vi "NIMS_NS_iir_notch.vi"(5 "Function name":string, 6 "Line number":i32, 7 "Number of outputs requested":i32, 8 "error in (no error)":errorcluster, 11 "[A]":variant[](array[variant])) -> (0 "error out":errorcluster, 3 "[funct(A)]":variant[](array[variant]))   [LabVIEW 2017]
uses:
  <vilib>/imath/engines/lvmath/Functions/Error Handling/error.ctl
  <instcachedir>/0/NIMS_RunTimeType_From StrictType (excl LVString)_1019F277F0A747EDBCA0F6C52CA54500.lvgen/NIMS_RunTimeType_From StrictType (excl LVString)_1019F277F0A747EDBCA0F6C52CA54500_000.vi
  <instcachedir>/0/NIMS_Get Scalar_w Error_1987D997E87247DDAC16EA23A5E9E4FC.lvgen/NIMS_Get Scalar_w Error_1987D997E87247DDAC16EA23A5E9E4FC_003.vi
  <instcachedir>/0/NIMS_Complex To Real_BE01396FDE034E8E94CEBBA1E368668D.lvgen/NIMS_Complex To Real_BE01396FDE034E8E94CEBBA1E368668D_000.vi
  <instcachedir>/0/NIMS_RunTimeType_To Numeric_1CBDAFC4EFAD4045A1DE52278D16738D.lvgen/NIMS_RunTimeType_To Numeric_1CBDAFC4EFAD4045A1DE52278D16738D_000.vi
  <vilib>/addons/Digital Filter Design/NI_DigFilter_MathScript.lvlib
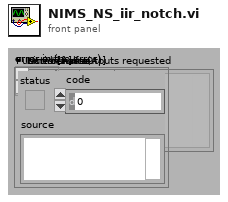
[diagram p1: front panel]
types:
  T1 = typedef "error.ctl" = enum16{"No Error", "Problem", "Input type must not be void", "Incorrect number of parameters", "Function not defined for non-numeric types", "An output variable of the user-defined function is undefined", "Function only defined for character arrays", "Function not defined for boolean, character, or single precision", "Function not defined for complex types", "Not a valid operation", "Inputs must be scalar", "Input matrices are not the same size", "Function only available on RT", "Input matrices must be nonnegative integers of the same type", "Arguments must be non-negative integers less than bitmax", "Number to complement must be less than 2^N", "Bit to get is outside range", "Bit to set is outside range", "Input must be real type ", "At least one parameter must be scalar", "Unable to display plug-in data on RT", "Function not defined for higher dimensional matrices", "Invalid attributes", "Wrong Type of Input Arguments", "Wrong Argument Option", "Invalid file identifier", "Indices must be real positive integers", "The variable is not a matrix data type.", "Number of elements must be the same for indices and values", "You cannot replace elements of a matrix with non-matrix data types.", "Cannot resize a 2D matrix with a linear index", "Unknown variable or symbol", "Indices out of range", "Empty matrix deletion can not be used with two indices", "Number of rows and columns must be the same for indices and values.", "Complex cannot be converted to Boolean", "Char cannot be converted to Boolean", "int64 cannot be converted to Boolean", "uint64 cannot be converted to Boolean", "You cannot convert a Boolean to a character.", "Incompatible input size in 3D surface function", "All rows must have the same number of columns", "Incompatible types", "Invalid matrix dimensions", "Dimension must be 1 or 2", "Base must be an integer between 2 and 36", "Invalid input", "Square matrix required", "Function 'timerstart' must be called before 'timerstop'", "Arguments must be positive real", "Step must not be zero", "Wrong number of input arguments", "Wrong number of output arguments", "Too many index arguments", "Input scalar must be >= 0", "Input scalar must be positive", "Input scalar must not be 0", "Input scalar must be in range [0,1]", "Can't use conditionally defined variable that's undefined", "Input must be a vector", "RT Exec Trace Toolkit not licensed", "Empty vector error", "All elements must be in domain [-1,1]", "All real elements of input vector must be >= 0", "All elements of input vector must be positive", "Values of input vectors are not compatible", "DAQmx not installed", "Input vector must be an increasing vector", "Dereferenced field does not exist within the struct", "A vector or matrix of structures must be indexed before it can be dereferenced", "Lenths of two input vectors are not compatible", "Invalid fieldname", "Empty matrix error", "Cannot use '.' on a type other than Struct", "Unused074", "Data type of the struct's field name is invalid", "Using . to dereference data that is not a struct", "Input struct contains invalid type ", "Size of input matrix is incompatible with input size", "Invalid format specifier", "Could not find field within struct", "Bad permutation array", "Mismatched fieldnames", "ode: User Function could not be opened", "ode: User Function signature does not meet ode requirements", "Unused085", "RunTime: MathScript could not be compiled", "Unknown function", "Only scalars and strings supported", "ode: User Function signature has incorrect number of inputs", "ode:User Function signature has incorrect number of outputs", "Range is too large", "End used without variable", "Function not available (RTE)", "Custom user error", "Arguments must be integers less than bitmax", "Shared library not found", "Header file not found", "Shared library already loaded", "Shared library not loaded", "Shared library function not found", "Shared library string return problem", "Problem calling shared library function", "Problem loading shared library from OS", "Problem parsing shared library header file", "Shared library incompatible types", "Shared library unsupported return type", "Shared library function not exported", "Shared library unsupported input type", "Problem unloading shared library from OS", "Function only available from UI", "Function specified in argument is missing", "An internal error has occurred", "Invalid object", "Invalid property", "Read-only property", "A break command has occurred", "A continue command has occurred", "A return command has occurred", "ode: times parameter invalid", "Function specified in argument has incorrect signature", "Function not found in file", "Reserved keyword cannot be defined as variable", "Reserved keyword cannot be defined as a function or script", "Arguments must be string literals", "Function not supported on this platform", "All columns must have the same number of rows", "Function ignored in RTE warning", "Cannot use : as a parameter that is not a variable", "Output can't be coerced to requested type", "Function not supported on current target", "Variable dependent on an unwired function input", "Unused132", "Unused133", "Unused134", "Unused135", "Unused136", "Unused137", "Unused138", "Unused139", "Global/Persistent must only take constants as arguments.", "Varargin must be last input in the function definition.", "Varargout must be last output in the function definition.", "Invalid output type. Cannot output a cell array of any type other than string.", "Invalid output type. Type is a dynamic struct.", "Invalid output type. Type is a struct that has a field whose type is not known until run-time", "Invalid output type. Type is a struct that has a field which is a plot object.", "MathScript parser DLL missing", "MathScript requires LabVIEW Full", "MathScript license is invalid or missing", "Varargout not supported except in assignments."}
  T2 = typedef "NIMS_CH_character datatype.ctl" = cluster{"Numeric":u8}
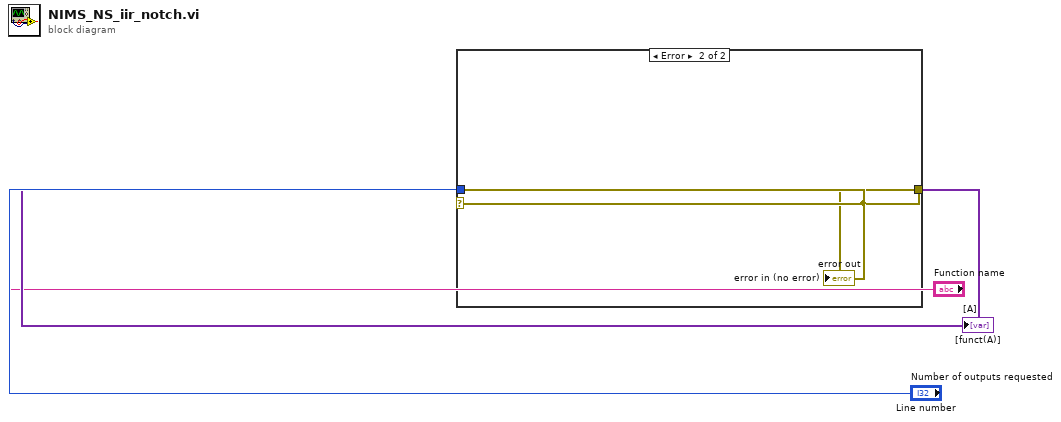
[diagram p0: block diagram]
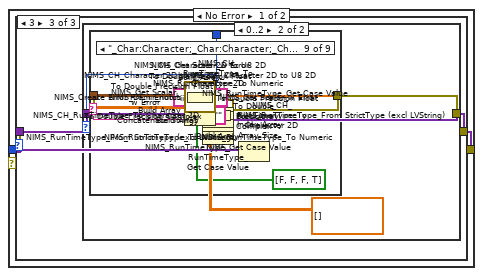
[diagram p2: hidden frame]
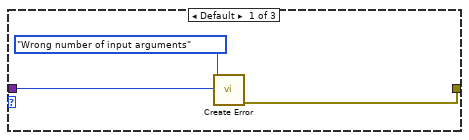
[diagram p3: hidden frame]
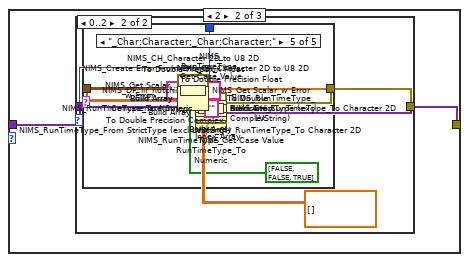
[diagram p4: hidden frame]
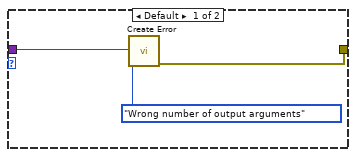
[diagram p5: hidden frame]
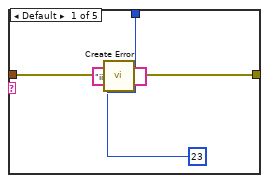
[diagram p6: hidden frame]
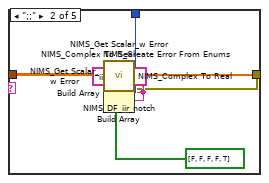
[diagram p7: hidden frame]
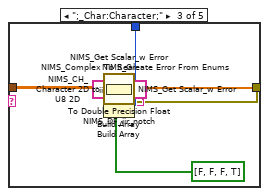
[diagram p8: hidden frame]
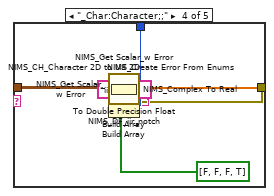
[diagram p9: hidden frame]
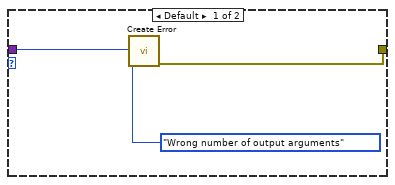
[diagram p10: hidden frame]
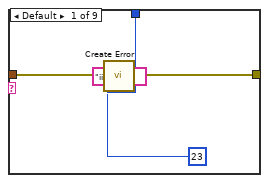
[diagram p11: hidden frame]
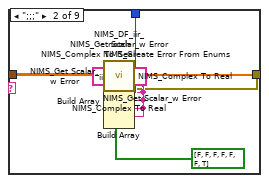
[diagram p12: hidden frame]
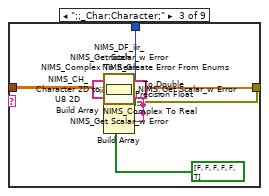
[diagram p13: hidden frame]
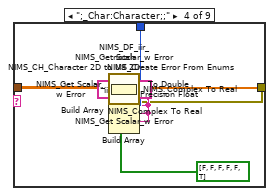
[diagram p14: hidden frame]
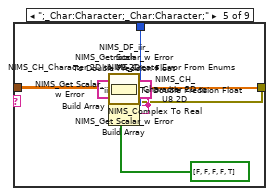
[diagram p15: hidden frame]
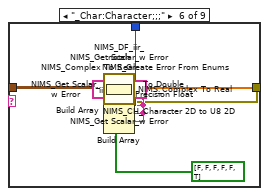
[diagram p16: hidden frame]
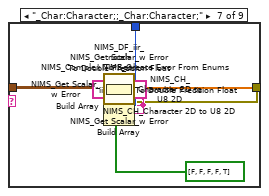
[diagram p17: hidden frame]
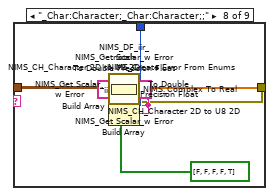
[diagram p18: hidden frame]
diagram:
  n1 = case shown="Error" "error in (no error)" {
    selector: "error in (no error)" -> [_ w404]
    tunnel: [w15 _] -> w4
    tunnel: [w14 w404] -> w3
    tunnel: "error in (no error)" -> [w13 _]
    tunnel: "Number of outputs requested" -> [w12 _]
    tunnel: "[A]" -> [w11 _]
    tunnel: "Function name" -> [w10 _]
    tunnel: "Line number" -> [w9 _]
    frame No Error {
      n2 = Array Size(array=w11) -> (size(s)=w8:i32)
      n3 = case shown="3" w8 {
        tunnel: [_ w27 w154] -> w15
        tunnel: w10 -> [w19 w24 w151]
        tunnel: w9 -> [w20 w25 w152]
        tunnel: w13 -> [w17 w23 w150]
        tunnel: [w16 w22 w149] -> w14
        tunnel: w12 -> [_ w21 w148]
        tunnel: w11 -> [_ w26 w153]
        frame Default {
          n4 = call <vilib>:"Create Error.vi"("Function name"=w19, "error in (no error)"=w17, "Error Enum"=error."Wrong number of input arguments", "Line number"=w20) -> ("error out"=w16:errorcluster)  [unwired: 6 in, 1 out]
        }
        frame 2 {
          n5 = case shown="0..2" w21 {
            tunnel: [_ w33] -> w27
            tunnel: w24 -> [w31 _]
            tunnel: w25 -> [w32 w57]
            tunnel: w23 -> [w29 w55]
            tunnel: [w28 w44] -> w22
            tunnel: w26 -> [_ w58]
            frame Default {
              n6 = call <vilib>:"Create Error.vi"("Function name"=w31, "error in (no error)"=w29, "Error Enum"=error."Wrong number of output arguments", "Line number"=w32) -> ("error out"=w28:errorcluster)  [unwired: 6 in, 1 out]
            }
            frame 0..2 {
              n7 = Index Array(array=w58) -> (element #1=w54:variant, element #2=w49:variant)  [unwired: 2 in]
              n8 = call <vilib>:"NIMS_RunTimeType_Get Case Value.vi"("Data In"=w49) -> ("Case Value"=w45:string)  [unwired: 9 in, 1 out]
              n9 = call <vilib>:"NIMS_CH_RunTimeType_To Character 2D.vi"("Variant"=w49) -> ("data"=w46:T2[][])  [unwired: 1 in]
              n10 = call-generic <vilib>:"NIMS_RunTimeType_To Numeric.vi"("DataType"=cdb[][] [], "Variant"=w49) -> ("data"=w47:cdb[][])  [unwired: 1 in]
              n11 = call <vilib>:"NIMS_RunTimeType_Get Case Value.vi"("Data In"=w54) -> ("Case Value"=w50:string)  [unwired: 9 in, 1 out]
              n12 = call <vilib>:"NIMS_CH_RunTimeType_To Character 2D.vi"("Variant"=w54) -> ("data"=w51:T2[][])  [unwired: 1 in]
              n13 = call-generic <vilib>:"NIMS_RunTimeType_To Numeric.vi"("DataType"=cdb[][] [], "Variant"=w54) -> ("data"=w52:cdb[][])  [unwired: 1 in]
              n14 = Concatenate Strings(w50, w45) -> (w56:string)
              n15 = case shown="\"_Char:Character;_Char:Character;\"" w56 {
                tunnel: w55 -> [w60 w70 w91 w112 w133]
                tunnel: [_ w65 w86 w107 w128] -> w43
                tunnel: [_ w64 w85 w106 w127] -> w39
                tunnel: [w59 w66 w87 w108 w129] -> w44
                tunnel: w52 -> [_ w83 w104 _ _]
                tunnel: w51 -> [_ _ _ w125 w146]
                tunnel: w47 -> [_ w80 _ w121 _]
                tunnel: w46 -> [_ _ w101 _ w142]
                tunnel: w57 -> [w63 w73 w94 w115 w136]
                frame Default {
                  n16 = call <vilib>:"Create Error.vi"("Function name"="iir_notch", "error in (no error)"=w60, "Error Enum"=23, "Line number"=w63) -> ("error out"=w59:errorcluster)  [unwired: 6 in, 1 out]
                }
                frame ";;" {
                  w68 = "iir_notch"
                  n17 = call-generic <vilib>:"NIMS_Complex To Real.vi"("A"=w80) -> ("Error Enum"=w76:T1, "Real(A)"=w79:dbl[][])  [unwired: 8 in, 1 out]
                  n18 = call-generic <vilib>:"NIMS_Get Scalar_w Error.vi"("A"=w79) -> ("Error Enum"=w75:T1, "Scalar"=w81:dbl)  [unwired: 8 in, 1 out]
                  n19 = call-generic <vilib>:"NIMS_Complex To Real.vi"("A"=w83) -> ("Error Enum"=w78:T1, "Real(A)"=w82:dbl[][])  [unwired: 8 in, 1 out]
                  n20 = call-generic <vilib>:"NIMS_Get Scalar_w Error.vi"("A"=w82) -> ("Error Enum"=w77:T1, "Scalar"=w84:dbl)  [unwired: 8 in, 1 out]
                  n21 = call <vilib>:"NIMS_DF_iir_notch.vi"("bw"=w81, "w"=w84) -> ("error"=w74:i32, "a"=w64:dbl[], "b"=w65:dbl[])  [unwired: 7 in]
                  n22 = Build Array(w68, w68, w68, w68, "iir_notch") -> (w71:string[])
                  n23 = Build Array(w78, w77, w76, w75, w74) -> (w72:i32[])
                  n24 = call <vilib>:"NIMS_Create Error From Enums.vi"("Error Code"=bool[] [FALSE, FALSE, FALSE, FALSE, TRUE], "error in (no error)"=w70, "Line no"=w73, "Error Enums"=w72, "Function names"=w71) -> ("error out"=w66:errorcluster)  [unwired: 6 in]
                }
                frame ";_Char:Character;" {
                  w89 = "iir_notch"
                  n25 = call <vilib>:"NIMS_CH_Character 2D to U8 2D.vi"("Character 2D array"=w101) -> ("U8 2D array"=w100:u8[][])  [unwired: 10 in]
                  n26 = To Double Precision Float(number=w100) -> (double precision float=w99:dbl[][])
                  n27 = call-generic <vilib>:"NIMS_Get Scalar_w Error.vi"("A"=w99) -> ("Error Enum"=w96:T1, "Scalar"=w102:dbl)  [unwired: 8 in, 1 out]
                  n28 = call-generic <vilib>:"NIMS_Complex To Real.vi"("A"=w104) -> ("Error Enum"=w98:T1, "Real(A)"=w103:dbl[][])  [unwired: 8 in, 1 out]
                  n29 = call-generic <vilib>:"NIMS_Get Scalar_w Error.vi"("A"=w103) -> ("Error Enum"=w97:T1, "Scalar"=w105:dbl)  [unwired: 8 in, 1 out]
                  n30 = call <vilib>:"NIMS_DF_iir_notch.vi"("bw"=w102, "w"=w105) -> ("error"=w95:i32, "a"=w85:dbl[], "b"=w86:dbl[])  [unwired: 7 in]
                  n31 = Build Array(w89, w89, w89, "iir_notch") -> (w92:string[])
                  n32 = Build Array(w98, w97, w96, w95) -> (w93:i32[])
                  n33 = call <vilib>:"NIMS_Create Error From Enums.vi"("Error Code"=bool[] [FALSE, FALSE, FALSE, TRUE], "error in (no error)"=w91, "Line no"=w94, "Error Enums"=w93, "Function names"=w92) -> ("error out"=w87:errorcluster)  [unwired: 6 in]
                }
                frame "_Char:Character;;" {
                  w110 = "iir_notch"
                  n34 = call-generic <vilib>:"NIMS_Complex To Real.vi"("A"=w121) -> ("Error Enum"=w118:T1, "Real(A)"=w120:dbl[][])  [unwired: 8 in, 1 out]
                  n35 = call-generic <vilib>:"NIMS_Get Scalar_w Error.vi"("A"=w120) -> ("Error Enum"=w117:T1, "Scalar"=w122:dbl)  [unwired: 8 in, 1 out]
                  n36 = call <vilib>:"NIMS_CH_Character 2D to U8 2D.vi"("Character 2D array"=w125) -> ("U8 2D array"=w124:u8[][])  [unwired: 10 in]
                  n37 = To Double Precision Float(number=w124) -> (double precision float=w123:dbl[][])
                  n38 = call-generic <vilib>:"NIMS_Get Scalar_w Error.vi"("A"=w123) -> ("Error Enum"=w119:T1, "Scalar"=w126:dbl)  [unwired: 8 in, 1 out]
                  n39 = call <vilib>:"NIMS_DF_iir_notch.vi"("bw"=w122, "w"=w126) -> ("error"=w116:i32, "a"=w106:dbl[], "b"=w107:dbl[])  [unwired: 7 in]
                  n40 = Build Array(w110, w110, w110, "iir_notch") -> (w113:string[])
                  n41 = Build Array(w119, w118, w117, w116) -> (w114:i32[])
                  n42 = call <vilib>:"NIMS_Create Error From Enums.vi"("Error Code"=bool[] [FALSE, FALSE, FALSE, TRUE], "error in (no error)"=w112, "Line no"=w115, "Error Enums"=w114, "Function names"=w113) -> ("error out"=w108:errorcluster)  [unwired: 6 in]
                }
                frame "_Char:Character;_Char:Character;" {
                  w131 = "iir_notch"
                  n43 = call <vilib>:"NIMS_CH_Character 2D to U8 2D.vi"("Character 2D array"=w142) -> ("U8 2D array"=w141:u8[][])  [unwired: 10 in]
                  n44 = To Double Precision Float(number=w141) -> (double precision float=w140:dbl[][])
                  n45 = call-generic <vilib>:"NIMS_Get Scalar_w Error.vi"("A"=w140) -> ("Error Enum"=w138:T1, "Scalar"=w143:dbl)  [unwired: 8 in, 1 out]
                  n46 = call <vilib>:"NIMS_CH_Character 2D to U8 2D.vi"("Character 2D array"=w146) -> ("U8 2D array"=w145:u8[][])  [unwired: 10 in]
                  n47 = To Double Precision Float(number=w145) -> (double precision float=w144:dbl[][])
                  n48 = call-generic <vilib>:"NIMS_Get Scalar_w Error.vi"("A"=w144) -> ("Error Enum"=w139:T1, "Scalar"=w147:dbl)  [unwired: 8 in, 1 out]
                  n49 = call <vilib>:"NIMS_DF_iir_notch.vi"("bw"=w143, "w"=w147) -> ("error"=w137:i32, "a"=w127:dbl[], "b"=w128:dbl[])  [unwired: 7 in]
                  n50 = Build Array(w131, w131, "iir_notch") -> (w134:string[])
                  n51 = Build Array(w139, w138, w137) -> (w135:i32[])
                  n52 = call <vilib>:"NIMS_Create Error From Enums.vi"("Error Code"=bool[] [FALSE, FALSE, TRUE], "error in (no error)"=w133, "Line no"=w136, "Error Enums"=w135, "Function names"=w134) -> ("error out"=w129:errorcluster)  [unwired: 6 in]
                }
              }
              n53 = Build Array(w39) -> (w38:dbl[][])
              n54 = To Double Precision Complex(1:w38) -> (0:w37:cdb[][])
              n55 = call-generic <vilib>:"NIMS_RunTimeType_From StrictType (excl LVString).vi"("Plug-In Name"="", "Data In"=w37) -> ("Data Out"=w34:variant)  [unwired: 2 in]
              n56 = Build Array(w43) -> (w42:dbl[][])
              n57 = To Double Precision Complex(1:w42) -> (0:w41:cdb[][])
              n58 = call-generic <vilib>:"NIMS_RunTimeType_From StrictType (excl LVString).vi"("Plug-In Name"="", "Data In"=w41) -> ("Data Out"=w35:variant)  [unwired: 2 in]
              n59 = Build Array(w35, w34) -> (w33:variant[])
            }
          }
        }
        frame 3 {
          n60 = case shown="0..2" w148 {
            tunnel: [_ w160] -> w154
            tunnel: w151 -> [w158 _]
            tunnel: w152 -> [w159 w189]
            tunnel: w150 -> [w156 w187]
            tunnel: [w155 w171] -> w149
            tunnel: w153 -> [_ w190]
            frame Default {
              n61 = call <vilib>:"Create Error.vi"("Function name"=w158, "error in (no error)"=w156, "Error Enum"=error."Wrong number of output arguments", "Line number"=w159) -> ("error out"=w155:errorcluster)  [unwired: 6 in, 1 out]
            }
            frame 0..2 {
              n62 = Index Array(array=w190) -> (element #1=w186:variant, element #2=w181:variant, element #3=w176:variant)  [unwired: 3 in]
              n63 = call <vilib>:"NIMS_RunTimeType_Get Case Value.vi"("Data In"=w176) -> ("Case Value"=w172:string)  [unwired: 9 in, 1 out]
              n64 = call <vilib>:"NIMS_CH_RunTimeType_To Character 2D.vi"("Variant"=w176) -> ("data"=w173:T2[][])  [unwired: 1 in]
              n65 = call-generic <vilib>:"NIMS_RunTimeType_To Numeric.vi"("DataType"=cdb[][] [], "Variant"=w176) -> ("data"=w174:cdb[][])  [unwired: 1 in]
              n66 = call <vilib>:"NIMS_RunTimeType_Get Case Value.vi"("Data In"=w181) -> ("Case Value"=w177:string)  [unwired: 9 in, 1 out]
              n67 = call <vilib>:"NIMS_CH_RunTimeType_To Character 2D.vi"("Variant"=w181) -> ("data"=w178:T2[][])  [unwired: 1 in]
              n68 = call-generic <vilib>:"NIMS_RunTimeType_To Numeric.vi"("DataType"=cdb[][] [], "Variant"=w181) -> ("data"=w179:cdb[][])  [unwired: 1 in]
              n69 = call <vilib>:"NIMS_RunTimeType_Get Case Value.vi"("Data In"=w186) -> ("Case Value"=w182:string)  [unwired: 9 in, 1 out]
              n70 = call <vilib>:"NIMS_CH_RunTimeType_To Character 2D.vi"("Variant"=w186) -> ("data"=w183:T2[][])  [unwired: 1 in]
              n71 = call-generic <vilib>:"NIMS_RunTimeType_To Numeric.vi"("DataType"=cdb[][] [], "Variant"=w186) -> ("data"=w184:cdb[][])  [unwired: 1 in]
              n72 = Concatenate Strings(w182, w177, w172) -> (w188:string)
              n73 = case shown="\"_Char:Character;_Char:Character;_Char:Character;\"" w188 {
                tunnel: w187 -> [w192 w202 w228 w254 w280 w306 w332 w358 w384]
                tunnel: [_ w197 w223 w249 w275 w301 w327 w353 w379] -> w170
                tunnel: [_ w196 w222 w248 w274 w300 w326 w352 w378] -> w166
                tunnel: [w191 w198 w224 w250 w276 w302 w328 w354 w380] -> w171
                tunnel: w184 -> [_ w220 w246 w272 w298 _ _ _ _]
                tunnel: w183 -> [_ _ _ _ _ w324 w350 w376 w402]
                tunnel: w179 -> [_ w217 w243 _ _ w320 w346 _ _]
                tunnel: w178 -> [_ _ _ w269 w295 _ _ w372 w398]
                tunnel: w174 -> [_ w214 _ w265 _ w317 _ w368 _]
                tunnel: w173 -> [_ _ w240 _ w291 _ w343 _ w394]
                tunnel: w189 -> [w195 w205 w231 w257 w283 w309 w335 w361 w387]
                frame Default {
                  n74 = call <vilib>:"Create Error.vi"("Function name"="iir_notch", "error in (no error)"=w192, "Error Enum"=23, "Line number"=w195) -> ("error out"=w191:errorcluster)  [unwired: 6 in, 1 out]
                }
                frame ";;;" {
                  w200 = "iir_notch"
                  n75 = call-generic <vilib>:"NIMS_Complex To Real.vi"("A"=w214) -> ("Error Enum"=w208:T1, "Real(A)"=w213:dbl[][])  [unwired: 8 in, 1 out]
                  n76 = call-generic <vilib>:"NIMS_Get Scalar_w Error.vi"("A"=w213) -> ("Error Enum"=w207:T1, "Scalar"=w215:dbl)  [unwired: 8 in, 1 out]
                  n77 = call-generic <vilib>:"NIMS_Complex To Real.vi"("A"=w217) -> ("Error Enum"=w210:T1, "Real(A)"=w216:dbl[][])  [unwired: 8 in, 1 out]
                  n78 = call-generic <vilib>:"NIMS_Get Scalar_w Error.vi"("A"=w216) -> ("Error Enum"=w209:T1, "Scalar"=w218:dbl)  [unwired: 8 in, 1 out]
                  n79 = call-generic <vilib>:"NIMS_Complex To Real.vi"("A"=w220) -> ("Error Enum"=w212:T1, "Real(A)"=w219:dbl[][])  [unwired: 8 in, 1 out]
                  n80 = call-generic <vilib>:"NIMS_Get Scalar_w Error.vi"("A"=w219) -> ("Error Enum"=w211:T1, "Scalar"=w221:dbl)  [unwired: 8 in, 1 out]
                  n81 = call <vilib>:"NIMS_DF_iir_notch.vi"("ab"=w215, "bw"=w218, "w"=w221) -> ("error"=w206:i32, "a"=w196:dbl[], "b"=w197:dbl[])  [unwired: 6 in]
                  n82 = Build Array(w200, w200, w200, w200, w200, w200, "iir_notch") -> (w203:string[])
                  n83 = Build Array(w212, w211, w210, w209, w208, w207, w206) -> (w204:i32[])
                  n84 = call <vilib>:"NIMS_Create Error From Enums.vi"("Error Code"=bool[] [FALSE, FALSE, FALSE, FALSE, FALSE, FALSE, TRUE], "error in (no error)"=w202, "Line no"=w205, "Error Enums"=w204, "Function names"=w203) -> ("error out"=w198:errorcluster)  [unwired: 6 in]
                }
                frame ";;_Char:Character;" {
                  w226 = "iir_notch"
                  n85 = call <vilib>:"NIMS_CH_Character 2D to U8 2D.vi"("Character 2D array"=w240) -> ("U8 2D array"=w239:u8[][])  [unwired: 10 in]
                  n86 = To Double Precision Float(number=w239) -> (double precision float=w238:dbl[][])
                  n87 = call-generic <vilib>:"NIMS_Get Scalar_w Error.vi"("A"=w238) -> ("Error Enum"=w233:T1, "Scalar"=w241:dbl)  [unwired: 8 in, 1 out]
                  n88 = call-generic <vilib>:"NIMS_Complex To Real.vi"("A"=w243) -> ("Error Enum"=w235:T1, "Real(A)"=w242:dbl[][])  [unwired: 8 in, 1 out]
                  n89 = call-generic <vilib>:"NIMS_Get Scalar_w Error.vi"("A"=w242) -> ("Error Enum"=w234:T1, "Scalar"=w244:dbl)  [unwired: 8 in, 1 out]
                  n90 = call-generic <vilib>:"NIMS_Complex To Real.vi"("A"=w246) -> ("Error Enum"=w237:T1, "Real(A)"=w245:dbl[][])  [unwired: 8 in, 1 out]
                  n91 = call-generic <vilib>:"NIMS_Get Scalar_w Error.vi"("A"=w245) -> ("Error Enum"=w236:T1, "Scalar"=w247:dbl)  [unwired: 8 in, 1 out]
                  n92 = call <vilib>:"NIMS_DF_iir_notch.vi"("ab"=w241, "bw"=w244, "w"=w247) -> ("error"=w232:i32, "a"=w222:dbl[], "b"=w223:dbl[])  [unwired: 6 in]
                  n93 = Build Array(w226, w226, w226, w226, w226, "iir_notch") -> (w229:string[])
                  n94 = Build Array(w237, w236, w235, w234, w233, w232) -> (w230:i32[])
                  n95 = call <vilib>:"NIMS_Create Error From Enums.vi"("Error Code"=bool[] [FALSE, FALSE, FALSE, FALSE, FALSE, TRUE], "error in (no error)"=w228, "Line no"=w231, "Error Enums"=w230, "Function names"=w229) -> ("error out"=w224:errorcluster)  [unwired: 6 in]
                }
                frame ";_Char:Character;;" {
                  w252 = "iir_notch"
                  n96 = call-generic <vilib>:"NIMS_Complex To Real.vi"("A"=w265) -> ("Error Enum"=w260:T1, "Real(A)"=w264:dbl[][])  [unwired: 8 in, 1 out]
                  n97 = call-generic <vilib>:"NIMS_Get Scalar_w Error.vi"("A"=w264) -> ("Error Enum"=w259:T1, "Scalar"=w266:dbl)  [unwired: 8 in, 1 out]
                  n98 = call <vilib>:"NIMS_CH_Character 2D to U8 2D.vi"("Character 2D array"=w269) -> ("U8 2D array"=w268:u8[][])  [unwired: 10 in]
                  n99 = To Double Precision Float(number=w268) -> (double precision float=w267:dbl[][])
                  n100 = call-generic <vilib>:"NIMS_Get Scalar_w Error.vi"("A"=w267) -> ("Error Enum"=w261:T1, "Scalar"=w270:dbl)  [unwired: 8 in, 1 out]
                  n101 = call-generic <vilib>:"NIMS_Complex To Real.vi"("A"=w272) -> ("Error Enum"=w263:T1, "Real(A)"=w271:dbl[][])  [unwired: 8 in, 1 out]
                  n102 = call-generic <vilib>:"NIMS_Get Scalar_w Error.vi"("A"=w271) -> ("Error Enum"=w262:T1, "Scalar"=w273:dbl)  [unwired: 8 in, 1 out]
                  n103 = call <vilib>:"NIMS_DF_iir_notch.vi"("ab"=w266, "bw"=w270, "w"=w273) -> ("error"=w258:i32, "a"=w248:dbl[], "b"=w249:dbl[])  [unwired: 6 in]
                  n104 = Build Array(w252, w252, w252, w252, w252, "iir_notch") -> (w255:string[])
                  n105 = Build Array(w263, w262, w261, w260, w259, w258) -> (w256:i32[])
                  n106 = call <vilib>:"NIMS_Create Error From Enums.vi"("Error Code"=bool[] [FALSE, FALSE, FALSE, FALSE, FALSE, TRUE], "error in (no error)"=w254, "Line no"=w257, "Error Enums"=w256, "Function names"=w255) -> ("error out"=w250:errorcluster)  [unwired: 6 in]
                }
                frame ";_Char:Character;_Char:Character;" {
                  w278 = "iir_notch"
                  n107 = call <vilib>:"NIMS_CH_Character 2D to U8 2D.vi"("Character 2D array"=w291) -> ("U8 2D array"=w290:u8[][])  [unwired: 10 in]
                  n108 = To Double Precision Float(number=w290) -> (double precision float=w289:dbl[][])
                  n109 = call-generic <vilib>:"NIMS_Get Scalar_w Error.vi"("A"=w289) -> ("Error Enum"=w285:T1, "Scalar"=w292:dbl)  [unwired: 8 in, 1 out]
                  n110 = call <vilib>:"NIMS_CH_Character 2D to U8 2D.vi"("Character 2D array"=w295) -> ("U8 2D array"=w294:u8[][])  [unwired: 10 in]
                  n111 = To Double Precision Float(number=w294) -> (double precision float=w293:dbl[][])
                  n112 = call-generic <vilib>:"NIMS_Get Scalar_w Error.vi"("A"=w293) -> ("Error Enum"=w286:T1, "Scalar"=w296:dbl)  [unwired: 8 in, 1 out]
                  n113 = call-generic <vilib>:"NIMS_Complex To Real.vi"("A"=w298) -> ("Error Enum"=w288:T1, "Real(A)"=w297:dbl[][])  [unwired: 8 in, 1 out]
                  n114 = call-generic <vilib>:"NIMS_Get Scalar_w Error.vi"("A"=w297) -> ("Error Enum"=w287:T1, "Scalar"=w299:dbl)  [unwired: 8 in, 1 out]
                  n115 = call <vilib>:"NIMS_DF_iir_notch.vi"("ab"=w292, "bw"=w296, "w"=w299) -> ("error"=w284:i32, "a"=w274:dbl[], "b"=w275:dbl[])  [unwired: 6 in]
                  n116 = Build Array(w278, w278, w278, w278, "iir_notch") -> (w281:string[])
                  n117 = Build Array(w288, w287, w286, w285, w284) -> (w282:i32[])
                  n118 = call <vilib>:"NIMS_Create Error From Enums.vi"("Error Code"=bool[] [FALSE, FALSE, FALSE, FALSE, TRUE], "error in (no error)"=w280, "Line no"=w283, "Error Enums"=w282, "Function names"=w281) -> ("error out"=w276:errorcluster)  [unwired: 6 in]
                }
                frame "_Char:Character;;;" {
                  w304 = "iir_notch"
                  n119 = call-generic <vilib>:"NIMS_Complex To Real.vi"("A"=w317) -> ("Error Enum"=w312:T1, "Real(A)"=w316:dbl[][])  [unwired: 8 in, 1 out]
                  n120 = call-generic <vilib>:"NIMS_Get Scalar_w Error.vi"("A"=w316) -> ("Error Enum"=w311:T1, "Scalar"=w318:dbl)  [unwired: 8 in, 1 out]
                  n121 = call-generic <vilib>:"NIMS_Complex To Real.vi"("A"=w320) -> ("Error Enum"=w314:T1, "Real(A)"=w319:dbl[][])  [unwired: 8 in, 1 out]
                  n122 = call-generic <vilib>:"NIMS_Get Scalar_w Error.vi"("A"=w319) -> ("Error Enum"=w313:T1, "Scalar"=w321:dbl)  [unwired: 8 in, 1 out]
                  n123 = call <vilib>:"NIMS_CH_Character 2D to U8 2D.vi"("Character 2D array"=w324) -> ("U8 2D array"=w323:u8[][])  [unwired: 10 in]
                  n124 = To Double Precision Float(number=w323) -> (double precision float=w322:dbl[][])
                  n125 = call-generic <vilib>:"NIMS_Get Scalar_w Error.vi"("A"=w322) -> ("Error Enum"=w315:T1, "Scalar"=w325:dbl)  [unwired: 8 in, 1 out]
                  n126 = call <vilib>:"NIMS_DF_iir_notch.vi"("ab"=w318, "bw"=w321, "w"=w325) -> ("error"=w310:i32, "a"=w300:dbl[], "b"=w301:dbl[])  [unwired: 6 in]
                  n127 = Build Array(w304, w304, w304, w304, w304, "iir_notch") -> (w307:string[])
                  n128 = Build Array(w315, w314, w313, w312, w311, w310) -> (w308:i32[])
                  n129 = call <vilib>:"NIMS_Create Error From Enums.vi"("Error Code"=bool[] [FALSE, FALSE, FALSE, FALSE, FALSE, TRUE], "error in (no error)"=w306, "Line no"=w309, "Error Enums"=w308, "Function names"=w307) -> ("error out"=w302:errorcluster)  [unwired: 6 in]
                }
                frame "_Char:Character;;_Char:Character;" {
                  w330 = "iir_notch"
                  n130 = call <vilib>:"NIMS_CH_Character 2D to U8 2D.vi"("Character 2D array"=w343) -> ("U8 2D array"=w342:u8[][])  [unwired: 10 in]
                  n131 = To Double Precision Float(number=w342) -> (double precision float=w341:dbl[][])
                  n132 = call-generic <vilib>:"NIMS_Get Scalar_w Error.vi"("A"=w341) -> ("Error Enum"=w337:T1, "Scalar"=w344:dbl)  [unwired: 8 in, 1 out]
                  n133 = call-generic <vilib>:"NIMS_Complex To Real.vi"("A"=w346) -> ("Error Enum"=w339:T1, "Real(A)"=w345:dbl[][])  [unwired: 8 in, 1 out]
                  n134 = call-generic <vilib>:"NIMS_Get Scalar_w Error.vi"("A"=w345) -> ("Error Enum"=w338:T1, "Scalar"=w347:dbl)  [unwired: 8 in, 1 out]
                  n135 = call <vilib>:"NIMS_CH_Character 2D to U8 2D.vi"("Character 2D array"=w350) -> ("U8 2D array"=w349:u8[][])  [unwired: 10 in]
                  n136 = To Double Precision Float(number=w349) -> (double precision float=w348:dbl[][])
                  n137 = call-generic <vilib>:"NIMS_Get Scalar_w Error.vi"("A"=w348) -> ("Error Enum"=w340:T1, "Scalar"=w351:dbl)  [unwired: 8 in, 1 out]
                  n138 = call <vilib>:"NIMS_DF_iir_notch.vi"("ab"=w344, "bw"=w347, "w"=w351) -> ("error"=w336:i32, "a"=w326:dbl[], "b"=w327:dbl[])  [unwired: 6 in]
                  n139 = Build Array(w330, w330, w330, w330, "iir_notch") -> (w333:string[])
                  n140 = Build Array(w340, w339, w338, w337, w336) -> (w334:i32[])
                  n141 = call <vilib>:"NIMS_Create Error From Enums.vi"("Error Code"=bool[] [FALSE, FALSE, FALSE, FALSE, TRUE], "error in (no error)"=w332, "Line no"=w335, "Error Enums"=w334, "Function names"=w333) -> ("error out"=w328:errorcluster)  [unwired: 6 in]
                }
                frame "_Char:Character;_Char:Character;;" {
                  w356 = "iir_notch"
                  n142 = call-generic <vilib>:"NIMS_Complex To Real.vi"("A"=w368) -> ("Error Enum"=w364:T1, "Real(A)"=w367:dbl[][])  [unwired: 8 in, 1 out]
                  n143 = call-generic <vilib>:"NIMS_Get Scalar_w Error.vi"("A"=w367) -> ("Error Enum"=w363:T1, "Scalar"=w369:dbl)  [unwired: 8 in, 1 out]
                  n144 = call <vilib>:"NIMS_CH_Character 2D to U8 2D.vi"("Character 2D array"=w372) -> ("U8 2D array"=w371:u8[][])  [unwired: 10 in]
                  n145 = To Double Precision Float(number=w371) -> (double precision float=w370:dbl[][])
                  n146 = call-generic <vilib>:"NIMS_Get Scalar_w Error.vi"("A"=w370) -> ("Error Enum"=w365:T1, "Scalar"=w373:dbl)  [unwired: 8 in, 1 out]
                  n147 = call <vilib>:"NIMS_CH_Character 2D to U8 2D.vi"("Character 2D array"=w376) -> ("U8 2D array"=w375:u8[][])  [unwired: 10 in]
                  n148 = To Double Precision Float(number=w375) -> (double precision float=w374:dbl[][])
                  n149 = call-generic <vilib>:"NIMS_Get Scalar_w Error.vi"("A"=w374) -> ("Error Enum"=w366:T1, "Scalar"=w377:dbl)  [unwired: 8 in, 1 out]
                  n150 = call <vilib>:"NIMS_DF_iir_notch.vi"("ab"=w369, "bw"=w373, "w"=w377) -> ("error"=w362:i32, "a"=w352:dbl[], "b"=w353:dbl[])  [unwired: 6 in]
                  n151 = Build Array(w356, w356, w356, w356, "iir_notch") -> (w359:string[])
                  n152 = Build Array(w366, w365, w364, w363, w362) -> (w360:i32[])
                  n153 = call <vilib>:"NIMS_Create Error From Enums.vi"("Error Code"=bool[] [FALSE, FALSE, FALSE, FALSE, TRUE], "error in (no error)"=w358, "Line no"=w361, "Error Enums"=w360, "Function names"=w359) -> ("error out"=w354:errorcluster)  [unwired: 6 in]
                }
                frame "_Char:Character;_Char:Character;_Char:Character;" {
                  w382 = "iir_notch"
                  n154 = call <vilib>:"NIMS_CH_Character 2D to U8 2D.vi"("Character 2D array"=w394) -> ("U8 2D array"=w393:u8[][])  [unwired: 10 in]
                  n155 = To Double Precision Float(number=w393) -> (double precision float=w392:dbl[][])
                  n156 = call-generic <vilib>:"NIMS_Get Scalar_w Error.vi"("A"=w392) -> ("Error Enum"=w389:T1, "Scalar"=w395:dbl)  [unwired: 8 in, 1 out]
                  n157 = call <vilib>:"NIMS_CH_Character 2D to U8 2D.vi"("Character 2D array"=w398) -> ("U8 2D array"=w397:u8[][])  [unwired: 10 in]
                  n158 = To Double Precision Float(number=w397) -> (double precision float=w396:dbl[][])
                  n159 = call-generic <vilib>:"NIMS_Get Scalar_w Error.vi"("A"=w396) -> ("Error Enum"=w390:T1, "Scalar"=w399:dbl)  [unwired: 8 in, 1 out]
                  n160 = call <vilib>:"NIMS_CH_Character 2D to U8 2D.vi"("Character 2D array"=w402) -> ("U8 2D array"=w401:u8[][])  [unwired: 10 in]
                  n161 = To Double Precision Float(number=w401) -> (double precision float=w400:dbl[][])
                  n162 = call-generic <vilib>:"NIMS_Get Scalar_w Error.vi"("A"=w400) -> ("Error Enum"=w391:T1, "Scalar"=w403:dbl)  [unwired: 8 in, 1 out]
                  n163 = call <vilib>:"NIMS_DF_iir_notch.vi"("ab"=w395, "bw"=w399, "w"=w403) -> ("error"=w388:i32, "a"=w378:dbl[], "b"=w379:dbl[])  [unwired: 6 in]
                  n164 = Build Array(w382, w382, w382, "iir_notch") -> (w385:string[])
                  n165 = Build Array(w391, w390, w389, w388) -> (w386:i32[])
                  n166 = call <vilib>:"NIMS_Create Error From Enums.vi"("Error Code"=bool[] [FALSE, FALSE, FALSE, TRUE], "error in (no error)"=w384, "Line no"=w387, "Error Enums"=w386, "Function names"=w385) -> ("error out"=w380:errorcluster)  [unwired: 6 in]
                }
              }
              n167 = Build Array(w166) -> (w165:dbl[][])
              n168 = To Double Precision Complex(1:w165) -> (0:w164:cdb[][])
              n169 = call-generic <vilib>:"NIMS_RunTimeType_From StrictType (excl LVString).vi"("Plug-In Name"="", "Data In"=w164) -> ("Data Out"=w161:variant)  [unwired: 2 in]
              n170 = Build Array(w170) -> (w169:dbl[][])
              n171 = To Double Precision Complex(1:w169) -> (0:w168:cdb[][])
              n172 = call-generic <vilib>:"NIMS_RunTimeType_From StrictType (excl LVString).vi"("Plug-In Name"="", "Data In"=w168) -> ("Data Out"=w162:variant)  [unwired: 2 in]
              n173 = Build Array(w162, w161) -> (w160:variant[])
            }
          }
        }
      }
    }
    frame Error {
    }
  }
  "error out" <- w3
  "[funct(A)]" <- w4
